vi "VideoRecorder.vi"() -> ()   [LabVIEW 2010]
uses:
  <instrlib>/niHWS/nihws.llb/niHWS Open File Permissions ID.ctl
  <vilib>/DAQmx/read.llb/DAQmx Read (Analog 1D Wfm NChan NSamp).vi
  <vilib>/DAQmx/create/channels.llb/DAQmx Create Channel (AI-Voltage-Basic).vi
  <vilib>/DAQmx/configure/timing.llb/DAQmx Timing (Sample Clock).vi
  <vilib>/daqmx/miscellaneous.llb/DAQmx Fill In Error Info.vi
  <instrlib>/niHWS/nihws.llb/niHWS Write Analog WDT.vi
  <instrlib>/niHWS/nihws.llb/niHWS Write Analog DBL.vi
  <vilib>/vision/driver/NI_Vision_Acquisition_Software.lvlib
  C:/Program Files/National Instruments/LabVIEW 2010/resource/objmgr/imaqdx.rc
  <vilib>/ptbypt/NI_PtbyPt.lvlib
  C:/Program Files/National Instruments/LabVIEW 2010/resource/objmgr/daqmx.rc
panel:
  in  "Channel Names":string[](array[string])
  out "Ephys Recoding Signals":waveform(dbl)[](graph)
  in  "Recording channels":tag
  in  "Extra":bool=TRUE
  in  "Camera":string(combo)
  in  "Video Modes":string(combo)
  in  "Compressor":string(combo)
  in  "Selected Path for AVI":path
  in  "Rec":bool
  out "fps":dbl format="%#_2g"
  in  "% Quality":i32=-1
  in  "Start":bool
  in  "Display":bool
  out "Rec Time":dbl format="%#_3g"
  in  "stop":bool
  out "Image Out":T1(plugin-control)
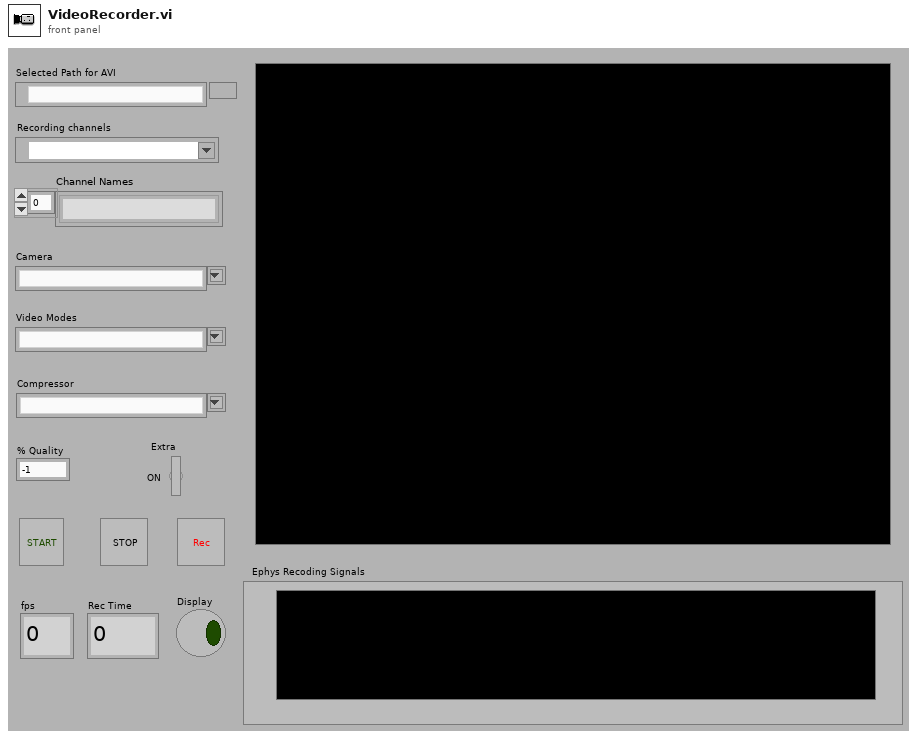
[diagram p1: front panel]
types:
  T1 = typedef "IMAQ Image.ctl" = refnum<image>
  T2 = typedef "niHWS Open File Permissions ID.ctl" = enum32{"Read Only", "Read/Write Existing", "Read/Write/Create New", "Read/Write/Create New Always"}
  T3 = cluster{"Type":u32, "Version":u32, "Flags":u32, "SerialNumberHigh":u32, "SerialNumberLow":u32, "BusType":u32, "InterfaceName":string, "VendorName":string, "ModelName":string, "CameraFileName":string, "CameraAttributeURL":string}[]
  T4 = cluster{"Type":u32, "Version":u32, "Flags":u32, "SerialNumberHigh":u32, "SerialNumberLow":u32, "BusType":u32, "InterfaceName":string, "VendorName":string, "ModelName":string, "CameraFileName":string, "CameraAttributeURL":string}
  T5 = typedef "IMAQdx.ctl" = refnum<k21>
  T6 = cluster{"Video Mode":u32, "Video Mode Name":string}[]
  T7 = typedef "AviRefnum.ctl" = refnum<k1>
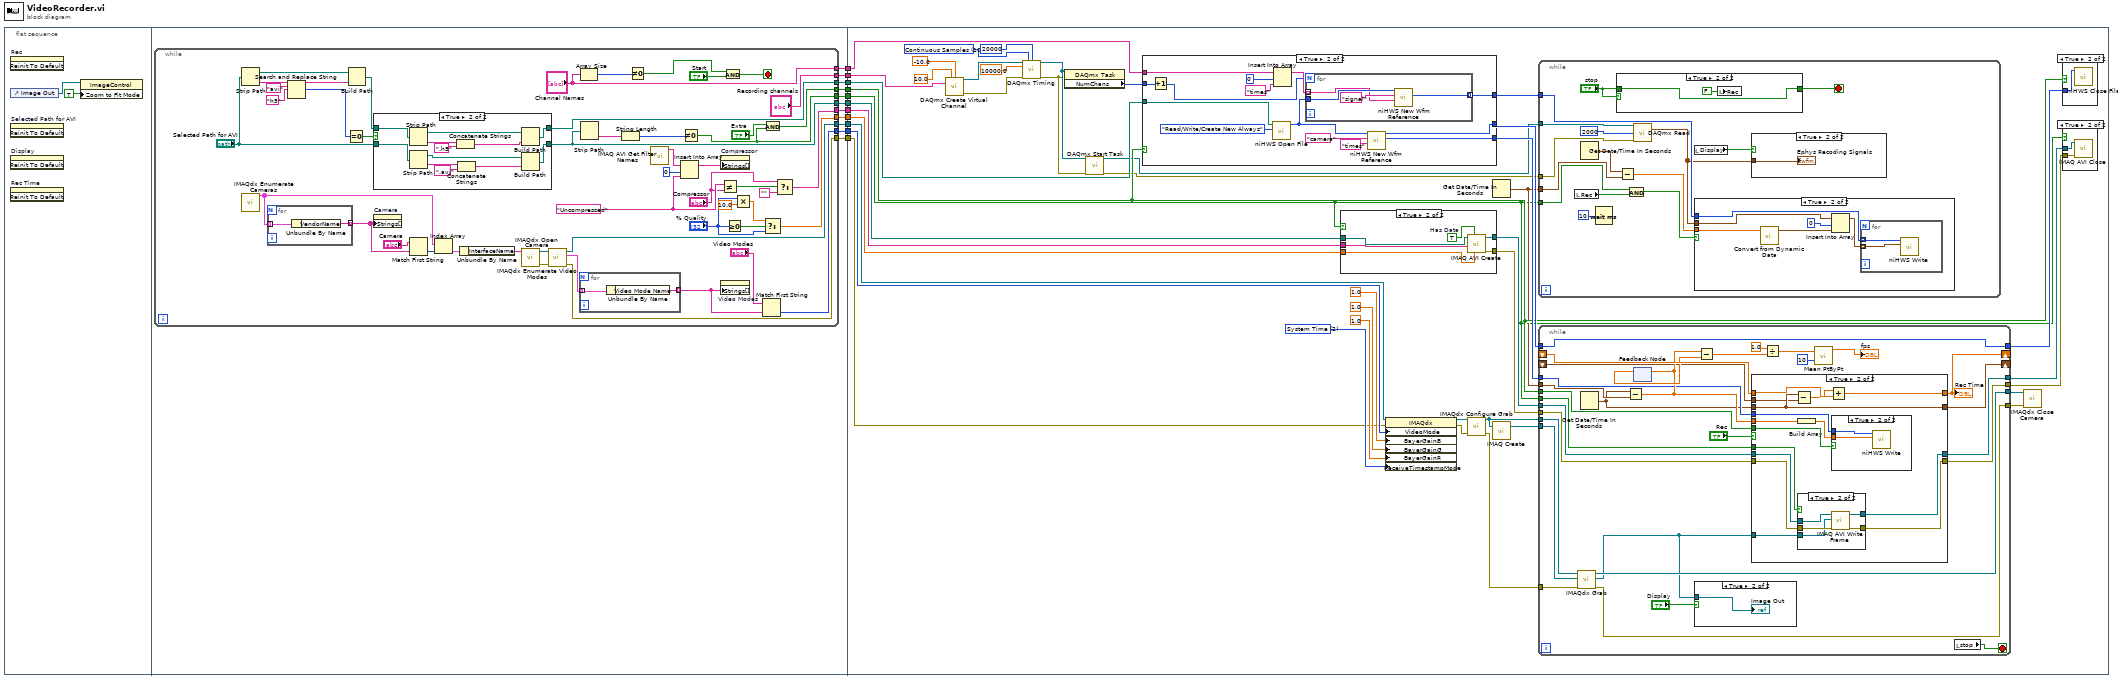
[diagram p0: block diagram]
diagram:
  n1 = flat-sequence {
    tunnel: [w24] -> w11
    tunnel: [w23] -> w10
    tunnel: [w22] -> w9
    tunnel: [w21] -> w8
    tunnel: [w20] -> w7
    tunnel: [w19] -> w6
    tunnel: [w18] -> w5
    tunnel: [w17] -> w4
    tunnel: [w16] -> w3
    tunnel: [w15] -> w2
    tunnel: [w14] -> w1
    tunnel: w11 -> [w123]
    tunnel: w10 -> [w117]
    tunnel: w9 -> [w122]
    tunnel: w8 -> [w121]
    tunnel: w7 -> [w110]
    tunnel: w6 -> [w115]
    tunnel: w5 -> [w111]
    tunnel: w4 -> [w109]
    tunnel: w3 -> [w92]
    tunnel: w2 -> [w100]
    tunnel: w1 -> [w96]
    frame #0 {
      n2 = invoke on="Rec" class="Bool (strict)" method="Reinit To Default"() -> ()  [unwired: 3 in, 3 out]
      n3 = control-ref of="Image Out"() -> (w13:refnum<vi>)
      n4 = invoke on="Selected Path for AVI" class="Path" method="Reinit To Default"() -> ()  [unwired: 3 in, 3 out]
      n5 = invoke on="Display" class="Bool (strict)" method="Reinit To Default"() -> ()  [unwired: 3 in, 3 out]
      n6 = invoke on="Rec Time" class="DigNum (strict)" method="Reinit To Default"() -> ()  [unwired: 3 in, 3 out]
      n7 = property on="Property Node" class="ImageControl"(reference=w13, "Zoom to Fit Mode"=TRUE) -> ()  [unwired: 1 in, 2 out]
    }
    frame #1 {
      n8 = while {
        tunnel: [w54] -> w24
        tunnel: [w68] -> w23
        tunnel: [w44] -> w22
        tunnel: [w61] -> w21
        tunnel: [w34] -> w20
        tunnel: [w37] -> w19
        tunnel: [w53] -> w18
        tunnel: [w31] -> w17
        tunnel: [w32] -> w16
        tunnel: ["Recording channels"] -> w15
        tunnel: ["Channel Names"] -> w14
        stop <- w25 stop-if-true
        w66 = "Uncompressed"
        n9 = Strip Path(path="Selected Path for AVI") -> (stripped path=w52:path, name=w50:string)
        n10 = call <vilib>:"IMAQdx Enumerate Cameras.vi"() -> ("Camera Information Array"=w57:T3)  [unwired: 10 in, 1 out]
        n11 = for {
          tunnel: w57 -> [w89] mode=indexing
          tunnel: [w88] -> w60 mode=indexing
          n12 = Unbundle By Name(w89) -> ("VendorName"=w88:string)
        }
        n13 = Search and Replace String(input string=w50, search string="avi", replace string="h5" ("replace string (\"\")")) -> (result string=w51:string, number of replacements=w40:i32)  [unwired: 5 in, 2 out]
        n14 = Equal To 0?(x=w40) -> (x = 0?=w39:bool)
        n15 = Build Path(base path=w52, name or relative path=w51) -> (appended path=w38:path)
        n16 = case shown="True" w39 {
          tunnel: "Selected Path for AVI" -> [w74 w87]
          tunnel: [w74 w86] -> w34
          tunnel: w38 -> [w75 w77]
          tunnel: [w75 w76] -> w37
          frame False {
          }
          frame True {
            n17 = Strip Path(path=w77) -> (stripped path=w81:path, name=w79:string)
            n18 = Strip Path(path=w87) -> (stripped path=w85:path, name=w83:string)
            n19 = Concatenate Strings(w79, ".h5" ("search string")) -> (w78:string)
            n20 = Concatenate Strings(w83, ".avi" ("search string")) -> (w82:string)
            n21 = Build Path(base path=w81, name or relative path=w78) -> (appended path=w76:path)
            n22 = Build Path(base path=w85, name or relative path=w82) -> (appended path=w86:path)
          }
        }
        n23 = property on="Camera" class="CmbBox"("Strings[]"=w60) -> ()  [unwired: 2 in, 2 out]
        n24 = Match First String(2:w60, 3:"Camera") -> (0:w58:i32)  [unwired: 1 out]
        n25 = Index Array(array=w57, index=w58) -> (element=w56:T4)
        n26 = Unbundle By Name(w56) -> ("InterfaceName"=w55:string)
        n27 = call <vilib>:"IMAQdx Open Camera.vi"("Session In"=w55) -> ("error out"=w72:errorcluster, "Session Out"=w73:T5)  [unwired: 9 in]
        n28 = call <vilib>:"IMAQdx Enumerate Video Modes.vi"("error in"=w72, "Session In"=w73) -> ("error out"=w53:errorcluster, "Video Modes"=w69:T6, "Session Out"=w54:T5)  [unwired: 6 in, 1 out]
        n29 = for {
          tunnel: w69 -> [w91] mode=indexing
          tunnel: [w90] -> w62 mode=indexing
          n30 = Unbundle By Name(w91) -> ("Video Mode Name"=w90:string)
        }
        n31 = Array Size(array="Channel Names") -> (size(s)=w28:i32)
        n32 = Strip Path(path=w34) -> (name=w35:string)  [unwired: 1 out]
        n33 = String Length(string=w35) -> (length=w36:i32)
        n34 = Not Equal To 0?(x=w28) -> (x != 0?=w27:bool)
        n35 = call "IMAQ AVI Get Filter Names"() -> ("Filter Names"=w42:string[])  [unwired: 10 in, 1 out]
        n36 = Insert Into Array(array=w42, index=0 ("Index"), new element=w66) -> (w70:string[])
        n37 = Not Equal To 0?(x=w36) -> (x != 0?=w32:bool)
        n38 = property on="Compressor" class="CmbBox"("Strings[]"=w70) -> ()  [unwired: 2 in, 2 out]
        n39 = Not Equal?(x=w66, y="Compressor") -> (x != y?=w64:bool)
        n40 = property on="Video Modes" class="CmbBox"("Strings[]"=w62) -> ()  [unwired: 2 in, 2 out]
        n41 = And(x=w27, y="Start") -> (x .and. y?=w25:bool)
        n42 = Greater Or Equal To 0?(x="% Quality") -> (x >= 0?=w46:bool)
        n43 = Multiply(x="% Quality", y=10.0) -> (x*y=w47:dbl)
        n44 = Match First String(2:w62, 3:"Video Modes") -> (0:w61:i32)  [unwired: 1 out]
        n45 = Select(t=w47, s=w46, f="% Quality") -> (s? t:f=w44:dbl)
        n46 = And(x="Extra", y=w32) -> (x .and. y?=w31:bool)
        n47 = Select(t="Compressor", s=w64, f="") -> (s? t:f=w68:string)
      }
    }
    frame #2 {
      w104 = 10123 items=["Finite Samples"=10178, "Continuous Samples"=10123, "Hardware Timed Single Point"=12522] ("sample mode")
      w116 = u32 2 items=["None", "Tick Count", "System Time"] ("ReceiveTimestampMode")
      n48 = call-poly <vilib>:"DAQmx Create Virtual Channel.vi"("maximum value"=10.0, "minimum value"=-10.0, "physical channels"=w100) -> ("task out"=w105:refnum<k21>, "error out"=w102:errorcluster)  [unwired: 11 in]
      n49 = call-poly <vilib>:"DAQmx Timing.vi"("task/channels in"=w105, "sample mode"=w104, "samples per channel"=20000, "rate"=10000.0, "error in"=w102) -> ("task out"=w95:refnum<k21>, "error out"=w94:errorcluster)  [unwired: 9 in]
      n50 = property class="DAQmx Task"(reference=w95, error in=w94) -> ("NumChans"=w93:u32)  [unwired: 2 out]
      n51 = call <vilib>:"DAQmx Start Task.vi"("task/channels in"=w95, "error in"=w94) -> ("task out"=w99:refnum<k21>, "error out"=w98:errorcluster)  [unwired: 12 in]
      n52 = case shown="True" w109 {
        tunnel: w115 -> [_ w181]
        tunnel: [_ w180] -> w114
        tunnel: [_ w179] -> w113
        tunnel: [_ w177] -> w108
        tunnel: w96 -> [_ w176]
        tunnel: w93 -> [_ w172]
        frame False {
        }
        frame True {
          n53 = Increment(x=w172) -> (x+1=w171:u32)
          n54 = call <instrlib>:"niHWS Open File.vi"("permissions (0:read only)"=niHWS_Open_File_Permissions_ID."Read/Write/Create New Always", "file path"=w181) -> ("file handle"=w178:u32)  [unwired: 8 in, 1 out]
          n55 = Insert Into Array(array=w176, index=0, new element="times" ("group name (empty)")) -> (w173:string[])
          n56 = for {
            N: w171 -> [_]
            tunnel: w178 -> [w187]
            tunnel: [w186] -> w177 mode=indexing
            tunnel: w173 -> [w185] mode=indexing
            n57 = call <instrlib>:"niHWS New Wfm Reference.vi"("waveform name (empty)"=w185, "group name (empty)"="signal", "file handle in"=w187) -> ("waveform reference"=w186:u32)  [unwired: 6 in, 2 out]
          }
          n58 = call <instrlib>:"niHWS New Wfm Reference.vi"("waveform name (empty)"="times" ("group name (empty)"), "group name (empty)"="camera", "file handle in"=w178) -> ("waveform reference"=w180:u32, "file handle out"=w179:u32)  [unwired: 6 in, 1 out]
        }
      }
      n59 = case shown="True" w92 {
        tunnel: [_ w168] -> w134
        tunnel: [_ w167] -> w131
        tunnel: w122 -> [_ w166]
        tunnel: w117 -> [_ w165]
        tunnel: w110 -> [_ w164]
        frame False {
        }
        frame True {
          w169 = TRUE  # Has Data
          n60 = call "IMAQ AVI Create"("quality"=w166, "Has Data"=w169, "Compression Filter"=w165, "AVI Path"=w164) -> ("error out"=w167:errorcluster, "Avi Refnum"=w168:T7)  [unwired: 3 in, 3 out]
        }
      }
      n61 = property class="IMAQdx"(reference=w123, error in=w111, "VideoMode"=w121, "BayerGainB"=1.0, "BayerGainG"=1.0, "BayerGainR"=1.0, "ReceiveTimestampMode"=w116) -> (reference out=w125:T5, error out=w124:errorcluster)
      n62 = call <vilib>:"IMAQdx Configure Grab.vi"("error in"=w124, "Session In"=w125) -> ("error out"=w129:errorcluster, "Session Out"=w120:T5)  [unwired: 8 in]
      n63 = Get Date/Time In Seconds() -> (seconds since 1Jan1904=w97:timestamp)
      n64 = call "IMAQ Create"("Image Name"=w120) -> ("New Image"=w130:T1)  [unwired: 4 in, 1 out]
      n65 = while {
        tunnel: w108 -> [w149]
        tunnel: w99 -> [w147]
        tunnel: w98 -> [w146]
        tunnel: w97 -> [w143]
        tunnel: w92 -> [w139]
        stop <- w135 stop-if-true
        n66 = local read "Rec"() -> (w138:bool)
        n67 = Get Date/Time In Seconds() -> (seconds since 1Jan1904=w144:timestamp)
        n68 = Wait (ms)(milliseconds to wait=u32 10) -> ()  [unwired: 1 out]
        n69 = case shown="True" "stop" {
          tunnel: "stop" -> [w150 w151]
          tunnel: [w150 w151] -> w135
          frame False {
          }
          frame True {
            n70 = local write "Rec"(FALSE ("Rec")) -> ()
          }
        }
        n71 = Subtract(x=w144, y=w143) -> (x-y=w142:dbl)
        n72 = And(x=w139, y=w138) -> (x .and. y?=w137:bool)
        n73 = call-poly <vilib>:"DAQmx Read.vi"("task/channels in"=w147, "number of samples per channel"=2000, "error in"=w146) -> ("data"=w145:waveform(dbl)[])  [unwired: 10 in, 2 out]
        n74 = local read "Display"() -> (w140:bool)
        n75 = case shown="True" w137 {
          tunnel: w149 -> [_ w159]
          tunnel: w145 -> [_ w157]
          tunnel: w142 -> [_ w158]
          frame False {
          }
          frame True {
            n76 = call "Convert from Dynamic Data"("Dynamic Data Type"=w158) -> ("Waveform"=w156:waveform(dbl))  [unwired: 3 in]
            n77 = Insert Into Array(array=w157, index=0, new element=w156) -> (w154:waveform(dbl)[])
            n78 = for {
              tunnel: w159 -> [w161] mode=indexing
              tunnel: w154 -> [w160] mode=indexing
              n79 = call-poly <instrlib>:"niHWS Write.vi"("analog waveform"=w160, "waveform reference in"=w161) -> ()  [unwired: 8 in, 2 out]
            }
          }
        }
        n80 = case shown="True" w140 {
          tunnel: w145 -> [_ w153]
          frame False {
          }
          frame True {
            "Ephys Recoding Signals" <- w153
          }
        }
      }
      n81 = while {
        tunnel: [w218] -> w133
        tunnel: [w217] -> w132
        tunnel: w134 -> [w216]
        tunnel: w131 -> [w215]
        tunnel: w130 -> [w214]
        tunnel: w120 -> [w213]
        tunnel: w129 -> [w212]
        tunnel: [w201] -> w119
        tunnel: [w209] -> w118
        shift-right: [w196] -> _
        shift-left: _ -> [w208]
        tunnel: w97 -> [w207]
        tunnel: w114 -> [w198]
        tunnel: w113 -> [w197]
        tunnel: [w197] -> w112
        shift-right: [w194] -> _
        shift-left: _ -> [w193]
        tunnel: w109 -> [w190]
        tunnel: w92 -> [w191]
        stop <- w189 stop-if-true
        n82 = call <vilib>:"IMAQdx Grab.vi"("error in"=w212, "Image In"=w214, "Session In"=w213) -> ("error out"=w209:errorcluster, "Image Out"=w200:T1, "Session Out"=w201:T5)  [unwired: 5 in, 1 out]
        n83 = Get Date/Time In Seconds() -> (seconds since 1Jan1904=w195:timestamp)
        n84 = Subtract(x=w195, y=w207) -> (x-y=w199:dbl)
        n85 = feedback-in #1(w199) -> ()
        n86 = feedback #1() -> (w206:dbl)  [unwired: 1 in]
        n87 = case shown="True" "Display" {
          tunnel: w200 -> [_ w245]
          frame False {
          }
          frame True {
            "Image Out" <- w245
          }
        }
        n88 = Subtract(x=w199, y=w206) -> (x-y=w204:dbl)
        n89 = case shown="True" "Rec" {
          tunnel: [w221 w237] -> w218
          tunnel: [w222 w236] -> w217
          tunnel: w216 -> [w221 w235]
          tunnel: w215 -> [w222 w234]
          tunnel: w200 -> [_ w233]
          tunnel: [w220 w228] -> w196
          tunnel: w208 -> [w220 w229]
          tunnel: w199 -> [_ w232]
          tunnel: w198 -> [_ w230]
          tunnel: [w219 w226] -> w194
          tunnel: w195 -> [w219 w226]
          tunnel: w193 -> [_ w225]
          tunnel: w190 -> [_ w224]
          tunnel: w191 -> [_ w223]
          frame False {
          }
          frame True {
            n90 = Subtract(x=w226, y=w225) -> (x-y=w227:dbl)
            n91 = Build Array(w232) -> (w231:dbl[])
            n92 = case shown="True" w223 {
              tunnel: [_ w242] -> w237
              tunnel: [_ w241] -> w236
              tunnel: w235 -> [_ w240]
              tunnel: w234 -> [_ w239]
              tunnel: w233 -> [_ w238]
              frame False {
              }
              frame True {
                n93 = call "IMAQ AVI Write Frame"("error in (no error)"=w239, "Image"=w238, "Avi Refnum"=w240) -> ("error out"=w241:errorcluster, "Avi Refnum (duplicate)"=w242:T7)  [unwired: 7 in]
              }
            }
            n94 = Add(x=w227, y=w229) -> (x+y=w228:dbl)
            n95 = case shown="True" w224 {
              tunnel: w231 -> [_ w244]
              tunnel: w230 -> [_ w243]
              frame False {
              }
              frame True {
                n96 = call-poly <instrlib>:"niHWS Write.vi"("data"=w244, "waveform reference in"=w243) -> ()  [unwired: 8 in, 2 out]
              }
            }
          }
        }
        "Rec Time" <- w196
        n97 = Divide(x=1.0, y=w204) -> (x/y=w203:dbl)
        n98 = call <vilib>:"Mean PtByPt.vi"("x"=w203, "sample length"=10) -> ("mean"=→"fps":dbl)  [unwired: 2 in, 1 out]
        n99 = local read "stop"() -> (w189:bool)
      }
      n100 = call <vilib>:"IMAQdx Close Camera.vi"("error in"=w118, "Session In"=w119) -> ()  [unwired: 9 in, 1 out]
      n101 = case shown="True" w109 {
        tunnel: w112 -> [_ w170]
        frame False {
        }
        frame True {
          n102 = call <instrlib>:"niHWS Close File.vi"("file handle"=w170) -> ()  [unwired: 10 in, 1 out]
        }
      }
      n103 = case shown="True" w92 {
        tunnel: w133 -> [_ w163]
        tunnel: w132 -> [_ w162]
        frame False {
        }
        frame True {
          n104 = call "IMAQ AVI Close"("error in (no error)"=w162, "Avi Refnum"=w163) -> ()  [unwired: 9 in, 1 out]
        }
      }
    }
  }
